vi "sinanju_getPos.vi"(0 "VISA资源名称":refnum<visa-resource-name>, 1 "错误输入（无错误）":errorcluster) -> (2 "VISA资源名称输出":refnum<visa-resource-name>, 3 "错误输出":errorcluster, 4 "值":sgl, 5 "值 2":sgl, 6 "值 3":sgl, 7 "值 4":sgl)   [LabVIEW 2017]
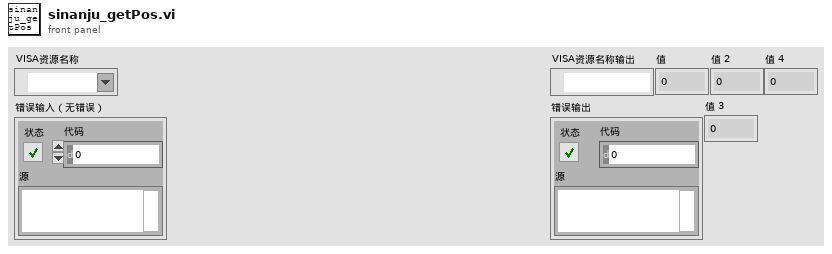
[diagram p1: front panel]
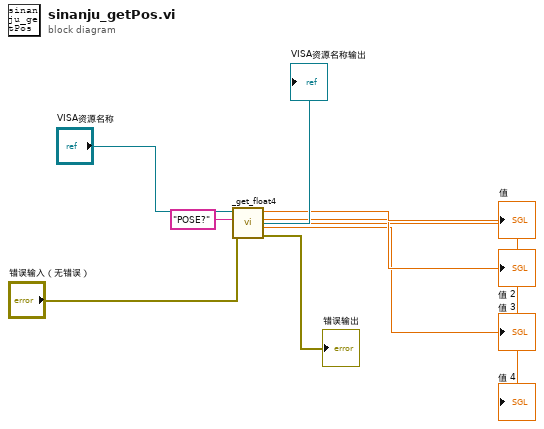
[diagram p0: block diagram]
diagram:
  n1 = call "_get_float4.vi"("错误输入（无错误）"="错误输入（无错误）", "写入缓冲区"="POSE?", "VISA资源名称"="VISA资源名称") -> ("错误输出"=→"错误输出":errorcluster, "值 3"=→"值 3":sgl, "值 2"=→"值 2":sgl, "值"=→"值":sgl, "值 4"=→"值 4":sgl, "VISA资源名称输出"=→"VISA资源名称输出":refnum<visa-resource-name>)  [unwired: 1 in]
